vi "Read TemplatesFolder Key.vi"(8 "Error In":errorcluster) -> (0 "Error Out":errorcluster, 3 "Templates Folder Path":string)   [LabVIEW 2021]
doc: "<add documentation here>"
uses:
  <vilib>/registry/registry.llb/Read Registry Value Simple STR.vi
panel:
  # "Development\nControls or indicators that are useful for development or testing, but which are not outputs of the VI."
  # "Input\nInputs to the VI"
  # "Output\nOutputs of the VI"
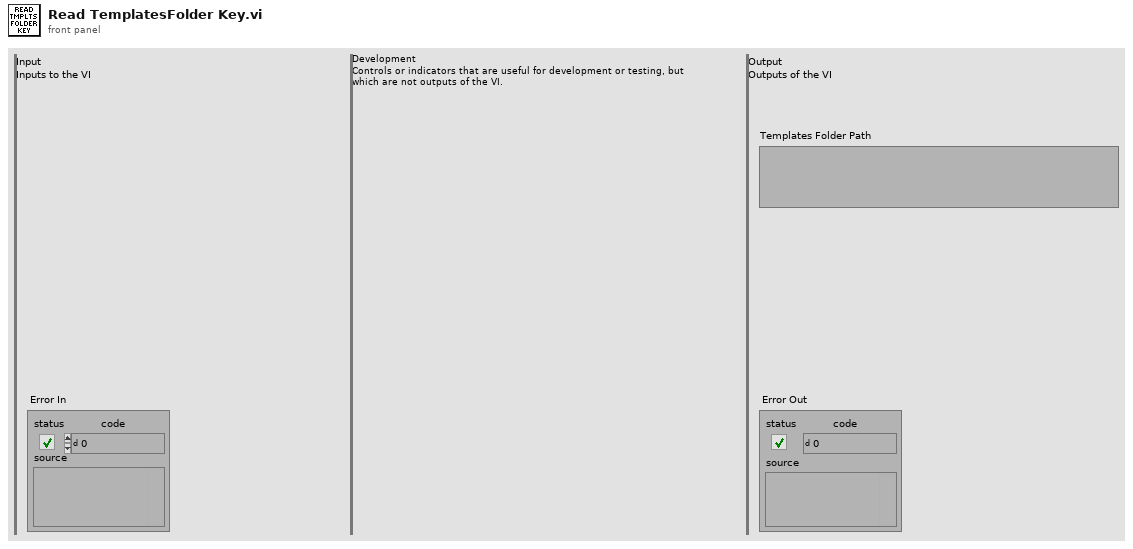
[diagram p1: front panel]
types:
  T1 = typedef "Registry RtKey.ctl" = enum32{"HKEY_CLASSES_ROOT", "HKEY_CURRENT_USER", "HKEY_LOCAL_MACHINE", "HKEY_USERS", "HKEY_PERFORMANCE_DATA", "HKEY_CURRENT_CONFIG", "HKEY_DYN_DATA"}
  T2 = typedef "Registry refnum.ctl" = refnum<k1>
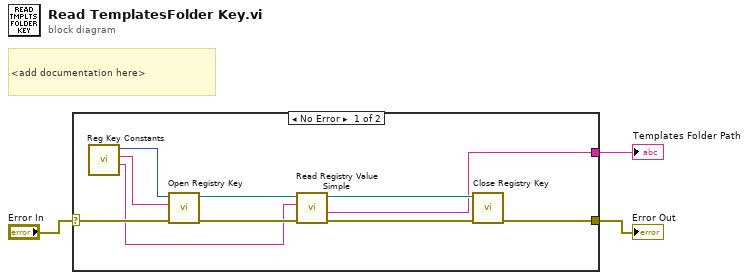
[diagram p0: block diagram]
diagram:
  # "<add documentation here>"
  n1 = case shown="No Error" "Error In" {
    selector: "Error In" -> [w13 w14]
    tunnel: [w10 w14] -> w2
    tunnel: [w7 _] -> w1
    frame No Error {
      n2 = call "Reg Key Constants.vi"() -> ("String Value Name"=w4:string, "Subkey Path"=w5:string, "Root Key"=w6:T1)  [unwired: 4 in, 1 out]
      n3 = call <vilib>:"Open Registry Key.vi"("error in (no error)"=w13, "subkey"=w5, "root key (HKEY_LOCAL_MACHINE)"=w6) -> ("error out"=w12:errorcluster, "refnum out"=w8:T2)  [unwired: 7 in]
      n4 = call-poly <vilib>:"Read Registry Value Simple.vi"("error in (no error)"=w12, "value"=w4, "refnum"=w8) -> ("error out"=w11:errorcluster, "String/Binary data"=w7:string, "refnum out"=w9:T2)  [unwired: 3 in, 1 out]
      n5 = call <vilib>:"Close Registry Key.vi"("error in (no error)"=w11, "refnum"=w9) -> ("error out"=w10:errorcluster)  [unwired: 5 in]
    }
    frame Error {
    }
  }
  "Error Out" <- w2
  "Templates Folder Path" <- w1
